vi "Zadanie 6 prodżekt.vi"() -> ()   [LabVIEW 2020]
panel:
  out "PWM":dbl[](graph)
  out "?":dbl(slide) scale=0.0..225.0
  in  "Numer":i32
  in  "stop":bool
  in  "Impuls":bool
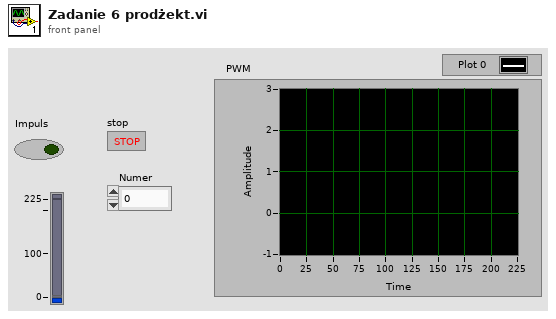
[diagram p1: front panel]
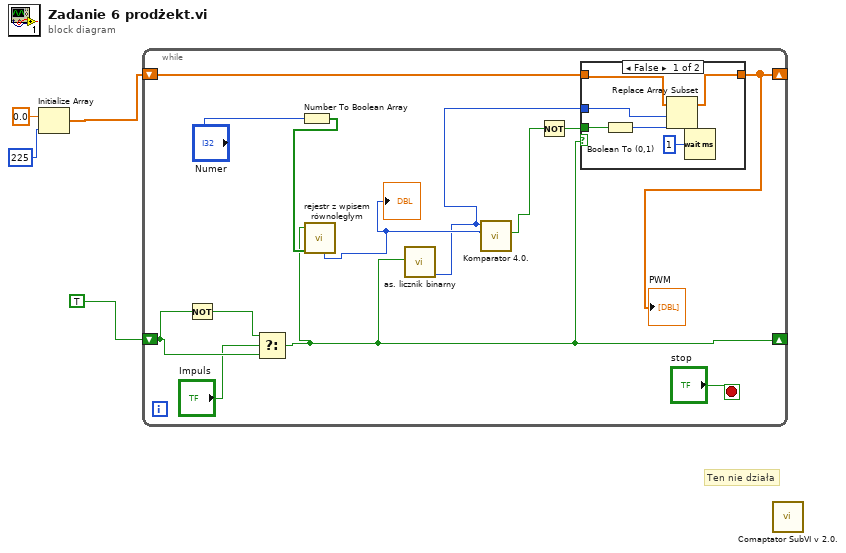
[diagram p0: block diagram]
diagram:
  # "Ten nie działa"
  n1 = Initialize Array(0.0 ("element"), 225 ("dimension size")) -> (w1:dbl[])
  n2 = while {
    shift-right: [w10] -> _
    shift-left: TRUE -> [w15]
    shift-right: [w5] -> _
    shift-left: w1 -> [w12]
    stop <- "stop" stop-if-true
    n3 = Not(x=w15) -> (.not. x?=w14:bool)
    n4 = Select(t=w14, s="Impuls", f=w15) -> (s? t:f=w10:bool)
    n5 = Number To Boolean Array(number="Numer") -> (Boolean array=w11:bool[])
    n6 = call "rejestr z wpisem równoległym.vi"("Wejście danych"=w11, "Switch"=w10) -> ("zliczenia wyjścia"=w8:u32)  [unwired: 7 in, 2 out]
    "?" <- w8
    n7 = call "as. licznik binarny.vi"("CP"=w10) -> ("ilość zliczeń"=w7:u32)  [unwired: 9 in, 1 out]
    n8 = call "Komparator 4.0..vi"("Q"=w8, "P"=w7) -> ("P>Q"=w6:bool)  [unwired: 8 in, 1 out]
    n9 = Not(x=w6) -> (.not. x?=w9:bool)
    n10 = case shown="False" w10 {
      tunnel: w9 -> [w23 _]
      tunnel: w7 -> [w21 _]
      tunnel: w12 -> [w20 w24]
      tunnel: [w19 w24] -> w5
      frame False {
        n11 = Boolean To (0,1)(Boolean=w23) -> (0, 1=w22:i16)
        n12 = Replace Array Subset(array=w20, new element=w22, index=w21) -> (w19:dbl[])
        n13 = Wait (ms)(milliseconds to wait=u32 1) -> ()  [unwired: 1 out]
      }
      frame True {
      }
    }
    "PWM" <- w5
  }
  n14 = call "Comaptator SubVI v 2.0..vi"() -> ()  [unwired: 10 in, 2 out]
